vi "read entry.vi"(8 "error in (no error)":errorcluster, 11 "id":string) -> (0 "error out":errorcluster, 1 "indices":i32[](array[numeric]), 2 "refnums":refnum<vi>[](array[refnum]), 3 "labels":string[](array[string]), 4 "plan sections":string[](array[string]), 6 "section settings":T1[][](array[typedef]))   [LabVIEW 2024, in "controls manager.lvlib"]
uses:
  controls manager.lvlib
  key value pair.ctl
  fgv actions.ctl
  <vilib>/Utility/error.llb/Error Cluster From Error Code.vi
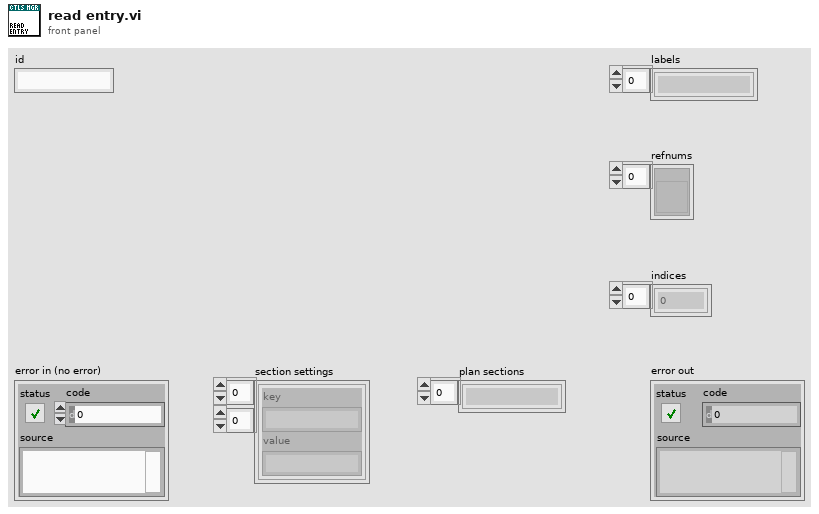
[diagram p1: front panel]
types:
  T1 = typedef "controls manager.lvlib/key value pair.ctl" = cluster{"key":string, "value":string}
  T2 = typedef "controls manager.lvlib/fgv actions.ctl" = enum16{"create", "get", "destroy"}
  T3 = typedef "controls manager.lvlib/collection type.ctl" = map{string, T4}
  T4 = typedef "controls manager.lvlib/entry type.ctl" = cluster{"controls":map{string, T5}, "plan":T6}
  T5 = typedef "controls manager.lvlib/control.ctl" = cluster{"refnum":refnum<vi>, "index":i32}
  T6 = typedef "controls manager.lvlib/controls plan.ctl" = map{string, T1[]}
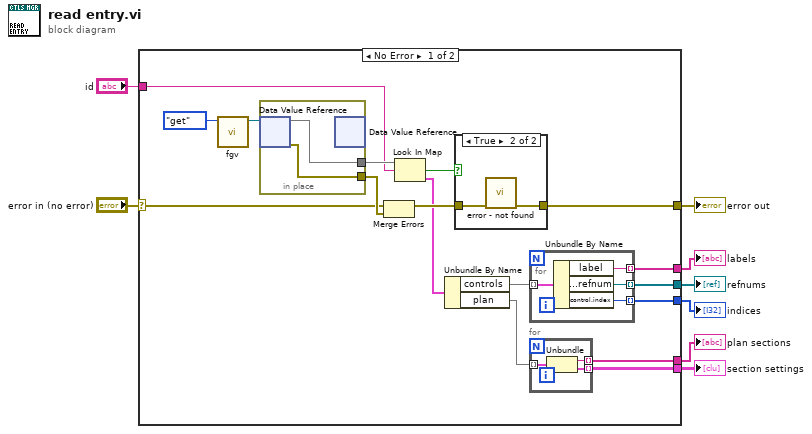
[diagram p0: block diagram]
diagram:
  n1 = case shown="No Error" "error in (no error)" {
    selector: "error in (no error)" -> [w21 w38]
    tunnel: [w17 w38] -> w7
    tunnel: "id" -> [w20 _]
    tunnel: [w15 _] -> w5
    tunnel: [w14 _] -> w4
    tunnel: [w11 _] -> w3
    tunnel: [w10 _] -> w2
    tunnel: [w9 _] -> w1
    frame No Error {
      n2 = call "fgv.vi"("action"=fgv_actions."get") -> ("dvr"=w24:refnum<data-value>)  [unwired: 9 in, 1 out]
      n3 = in-place {
        in-place-border: [w37] -> w25
        in-place-border: [w36] -> w22
        n4 = in-place-dvr #1(w24) -> (w37:T3, w36:errorcluster)
        n5 = in-place-dvr #1() -> ()  [unwired: 1 in, 2 out]
      }
      n6 = Merge Errors(w21, w22) -> (w18:errorcluster)
      n7 = Look In Map(map=w25, key=w20) -> (key not found?=w19:bool, value=w13:T4)  [unwired: 1 in]
      n8 = Unbundle By Name(w13) -> ("controls"=w12:map{string, T5}, "plan"=w16:T6)
      n9 = case shown="True" w19 {
        tunnel: w18 -> [w33 w35]
        tunnel: [w33 w34] -> w17
        frame False {
        }
        frame True {
          n10 = call "error - not found.vi"("error in (no error)"=w35) -> ("error out"=w34:errorcluster)  [unwired: 10 in]
        }
      }
      n11 = for {
        tunnel: w12 -> [w32] mode=indexing
        tunnel: [w31] -> w11 mode=indexing
        tunnel: [w30] -> w10 mode=indexing
        tunnel: [w29] -> w9 mode=indexing
        n12 = Unbundle By Name(w32) -> ("label"=w31:string, "control.refnum"=w30:refnum<vi>, "control.index"=w29:i32)
      }
      n13 = for {
        tunnel: w16 -> [w28] mode=indexing
        tunnel: [w27] -> w15 mode=indexing
        tunnel: [w26] -> w14 mode=indexing
        n14 = Unbundle(w28) -> ("section"=w27:string, "settings"=w26:T1[])
      }
    }
    frame Error {
    }
  }
  "error out" <- w7
  "labels" <- w3
  "refnums" <- w2
  "plan sections" <- w5
  "section settings" <- w4
  "indices" <- w1
